vi "niScope Fetch Array Measurement Cluster.vi"(0 "instrument handle":refnum<k15>, 1 "timeout":dbl=5.0 format="%.2f", 5 "channels":string="0", 7 "array measurement":T3=4000 items=["None"=4000, "Last Acq. Histogram"=4001, "Multi Acq. Voltage Histogram"=4004, "Multi Acq. Time Histogram"=4005, "Multi Acq. Average"=4016, "Polynomial Interpolation"=4011, "Array Integral"=4006, "Derivative"=4007, "Inverse"=4008, "Multiply Channels"=4012, "Add Channels"=4013, "Subtract Channels"=4014, "Divide Channels"=4015, "Array Offset"=4025, "Array Gain"=4026, "Hanning Window"=4009, "Flat Top Window"=4010, "Hamming Window"=4020, "Triangle Window"=4023, "Blackman Window"=4024, "FIR Windowed Filter"=4021, "Bessel IIR Filter"=4022, "Butterworth IIR Filter"=4017, "Chebyshev IIR Filter"=4018, "FFT Phase Spectrum"=4002, "FFT Amp. Spectrum (Volts RMS)"=4003, "FFT Amp. Spectrum (dB)"=4019], 11 "error in":errorcluster, 12 "meas waveform size":i32=-1) -> (4 "instrument handle out":refnum<k15>, 6 "meas wfm info":T1 {"reserved2" format="%.2f"; "reserved1" format="%.2f"; "offset" format="%^.3e"; "gain" format="%^.3e"; "xIncrement" format="%^.3e"; "relativeInitialX" format="%^.3e"; "absoluteInitialX" format="%^.3e"}, 10 "meas waveform":T2 {"measWfm" format="%.2f"; "xIncrement" format="%.2f"; "relativeInitialX" format="%.2f"}, 15 "error out":errorcluster)   [LabVIEW 2011]
doc: "Obtains a waveform from the digitizer and returns the specified measurement array for a single channel and record as a cluster along with timing data."
uses:
  <instrlib>/niScope/Controls/niScope array measurement.ctl
  niScope_32.dll
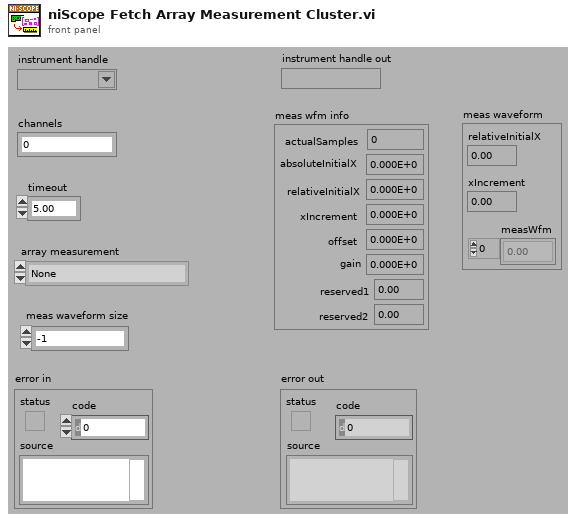
[diagram p1: front panel]
types:
  T1 = cluster{"actualSamples":i32, "absoluteInitialX":dbl, "relativeInitialX":dbl, "xIncrement":dbl, "offset":dbl, "gain":dbl, "reserved1":dbl, "reserved2":dbl}
  T2 = cluster{"relativeInitialX":dbl, "xIncrement":dbl, "measWfm":dbl[]}
  T3 = typedef "niScope array measurement.ctl" = i32
  T4 = cluster{"xIncrement":dbl, "xIncrement":dbl, "measWfm":dbl[]}
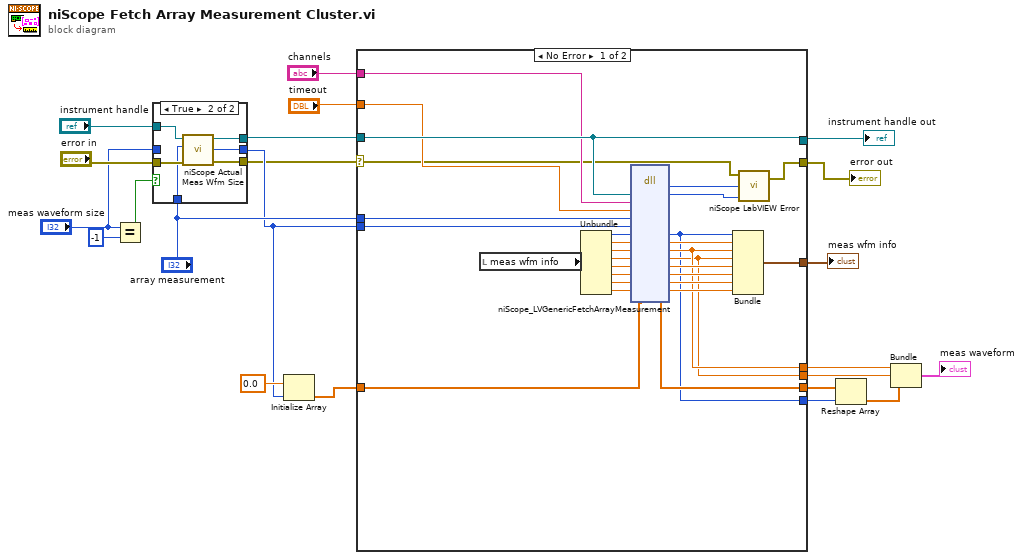
[diagram p0: block diagram]
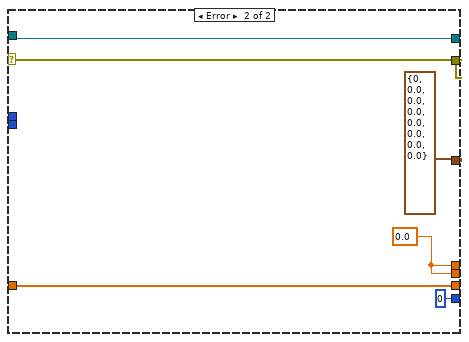
[diagram p3: hidden frame]
diagram:
  n1 = Equal?(x="meas waveform size", y=-1) -> (x = y?=w20:bool)
  n2 = case shown="True" w20 {
    tunnel: [w25 w31] -> w1
    tunnel: "error in" -> [w25 w30]
    tunnel: "instrument handle" -> [w24 w29]
    tunnel: [w24 w28] -> w15
    tunnel: [w23 w27] -> w5
    tunnel: "meas waveform size" -> [w23 _]
    tunnel: "array measurement" -> [_ w26]
    frame False {
    }
    frame True {
      n3 = call <instrlib>:"niScope Actual Meas Wfm Size.vi"("error in"=w30, "arrayMeasFunction"=w26, "instrument handle"=w29) -> ("error out"=w31:errorcluster, "meas wfm size"=w27:i32, "instrument handle out"=w28:refnum<k15>)  [unwired: 6 in]
    }
  }
  n4 = Initialize Array(0.0 ("Element Data"), w5) -> (w4:dbl[])
  n5 = case shown="No Error" w1 {
    selector: w1 -> [w32 w61]
    tunnel: [w60 w61] -> w22
    tunnel: w15 -> [w57 w66]
    tunnel: w5 -> [w53 _]
    tunnel: [w57 w66] -> w16
    tunnel: [w52 T1 {"actualSamples"=0, "absoluteInitialX"=0.0, "relativeInitialX"=0.0, "xIncrement"=0.0, "offset"=0.0, "gain"=0.0, "reserved1"=0.0, "reserved2"=0.0}] -> w13
    tunnel: "array measurement" -> [w49 _]
    tunnel: [w48 w62] -> w10
    tunnel: [w47 w62] -> w9
    tunnel: [w46 w64] -> w8
    tunnel: [w45 0 ("actualSamples")] -> w7
    tunnel: w4 -> [w44 w64]
    tunnel: "timeout" -> [w34 _]
    tunnel: "channels" -> [w33 _]
    frame No Error {
      n6 = local read "meas wfm info"() -> (w43:T1)
      n7 = Unbundle(w43) -> ("actualSamples"=w42:i32, "absoluteInitialX"=w41:dbl, "relativeInitialX"=w40:dbl, "xIncrement"=w39:dbl, "offset"=w38:dbl, "gain"=w37:dbl, "reserved1"=w36:dbl, "reserved2"=w35:dbl)
      n8 = dll-call lib="niScope_*.*" fn="niScope_LVGenericFetchArrayMeasurement"("instrument handle"=w57, "channel"=w33, "timeout"=w34, "arrayMeasFunction"=w49, "measWfmSize"=w53, "actualSamples"=w42, "absoluteInitialX"=w41, "relativeInitialX"=w40, "xIncrement"=w39, "offset"=w38, "gain"=w37, "reserved1"=w36, "reserved2"=w35, "measWfm"=w44) -> ("status"=w59:i32, "instrument handle"=w58:u32, "actualSamples"=w45:i32, "absoluteInitialX"=w54:dbl, "relativeInitialX"=w48:dbl, "xIncrement"=w47:dbl, "offset"=w55:dbl, "gain"=w56:dbl, "reserved1"=w51:dbl, "reserved2"=w50:dbl, "measWfm"=w46:dbl[])  [unwired: 7 in, 2 out]
      n9 = Bundle("actualSamples"=w45, "absoluteInitialX"=w54, "relativeInitialX"=w48, "xIncrement"=w47, "offset"=w55, "gain"=w56, "reserved1"=w51, "reserved2"=w50) -> (w52:T1)  [unwired: 1 in]
      n10 = call <instrlib>:"niScope LabVIEW Error.vi"("instrument handle"=w58, "niScope error code (0)"=w59, "error in (no error)"=w32) -> ("error out"=w60:errorcluster)  [unwired: 2 in]
    }
    frame Error {
      w62 = 0.0 ("xIncrement")
    }
  }
  "error out" <- w22
  "instrument handle out" <- w16
  "meas wfm info" <- w13
  n11 = Reshape Array(w8, w7) -> (w12:dbl[])
  n12 = Bundle("xIncrement"=w10, "xIncrement"=w9, "measWfm"=w12) -> (→"meas waveform":T4)  [unwired: 1 in]
